vi "Lidar Finder_OLD.vi"(3 "Stop":bool, 5 "VISA resource name":refnum<visa-resource-name>="Hukuyo") -> (0 "Objects":cluster{i32, i32}[](array[cluster]), 1 "Widest Object":cluster{i32, i32}, 2 "Where to Point":i32)   [LabVIEW 2014]
uses:
  <instrlib>/Hokuyo URG Series/Public/Initialize-Standard.vi
  <instrlib>/Hokuyo URG Series/Hokuyo URG Series.lvlib
panel:
  in  "Tab Control":enum32{"Raw Data", "Clean Data"}(tab)
  out "Data Aquired":picture
  out "Object Graph":i32[](graph)
  out "Edges":i32[](graph)
  out "Blinky LIDAR  Running":bool
  in  "polar attributes (hidden)":T1={"maximum"=30000.0, "minimum"=0.0, "clip to min"=FALSE, "log?(F)"=TRUE, "grid color"=6710886, "plot color"=65280, "fmt and prec"={"format"=enum."Decimal", "precision"=0}, "visible section"=8} {"minimum" format="%0.2f"; "maximum" format="%0.2f"}
  in  "Grid Color":u32(colorbox)=11776947
  in  "Plot Color":u32(colorbox)=14422272
  in  "Max (m)":dbl=1.0
  in  "End Point":dbl=40.0
  in  "Start Point":dbl=-50.0
  in  "Cluster Count":dbl=1.0
  in  "Encoding Width":u16(ring)=3 items=["2 Byte"=2, "3 Byte"=3]
  # "click here to run"
  # "Hokuyo LIDAR Example"
  # "Plot in mm"
  # "start at-50"
  # "start at 40"
  # "Start with 1.0 m"
  # "Hokuyo plugged in?"
  # "Location"
  # "Width"
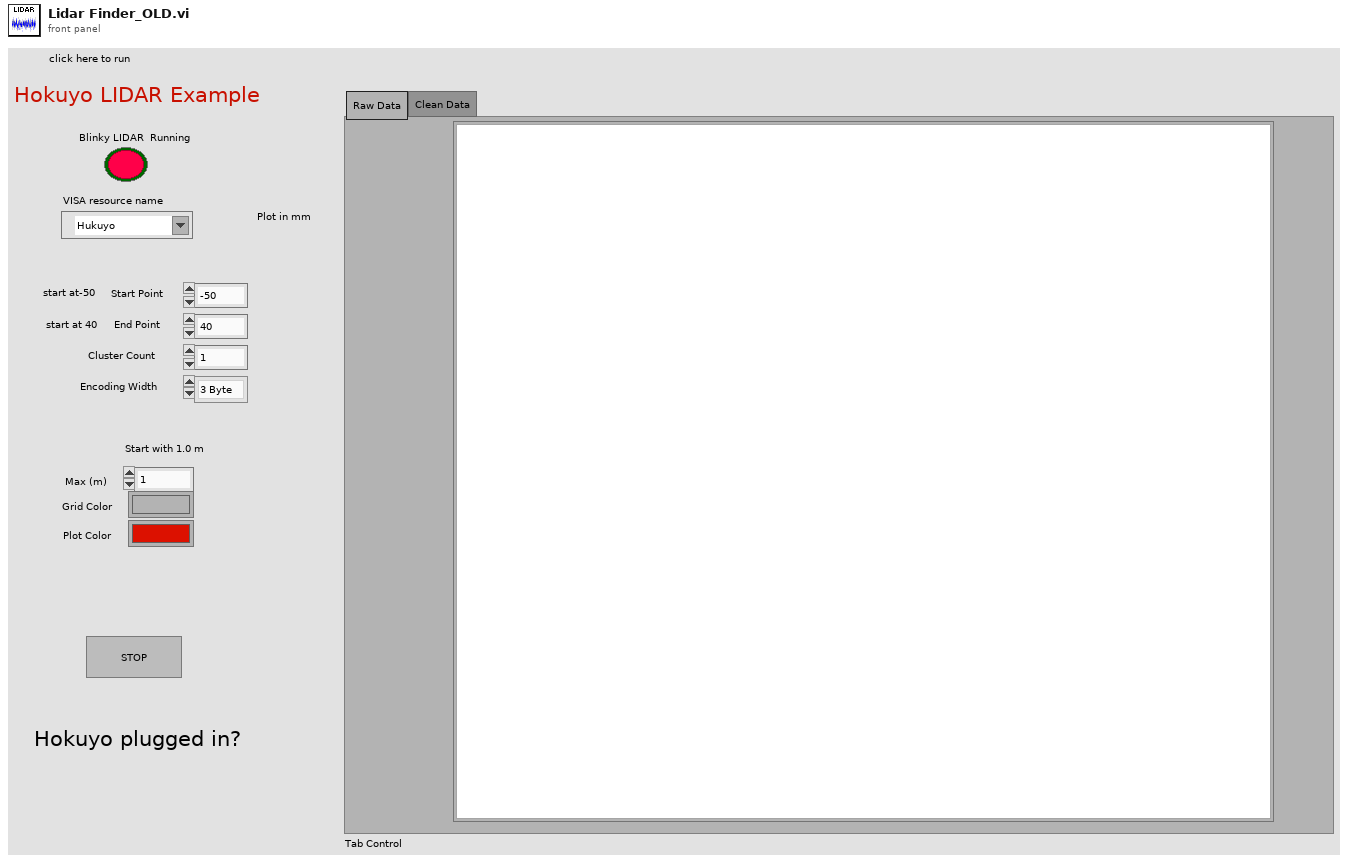
[diagram p1: front panel]
types:
  T1 = cluster{"maximum":dbl, "minimum":dbl, "clip to min":bool, "log?(F)":bool, "grid color":u32, "plot color":u32, "fmt and prec":cluster{"format":enum8{"Decimal", "Scientific", "Engineering", "Binary", "Octal", "Hex"}, "precision":u8}, "visible section":u16}
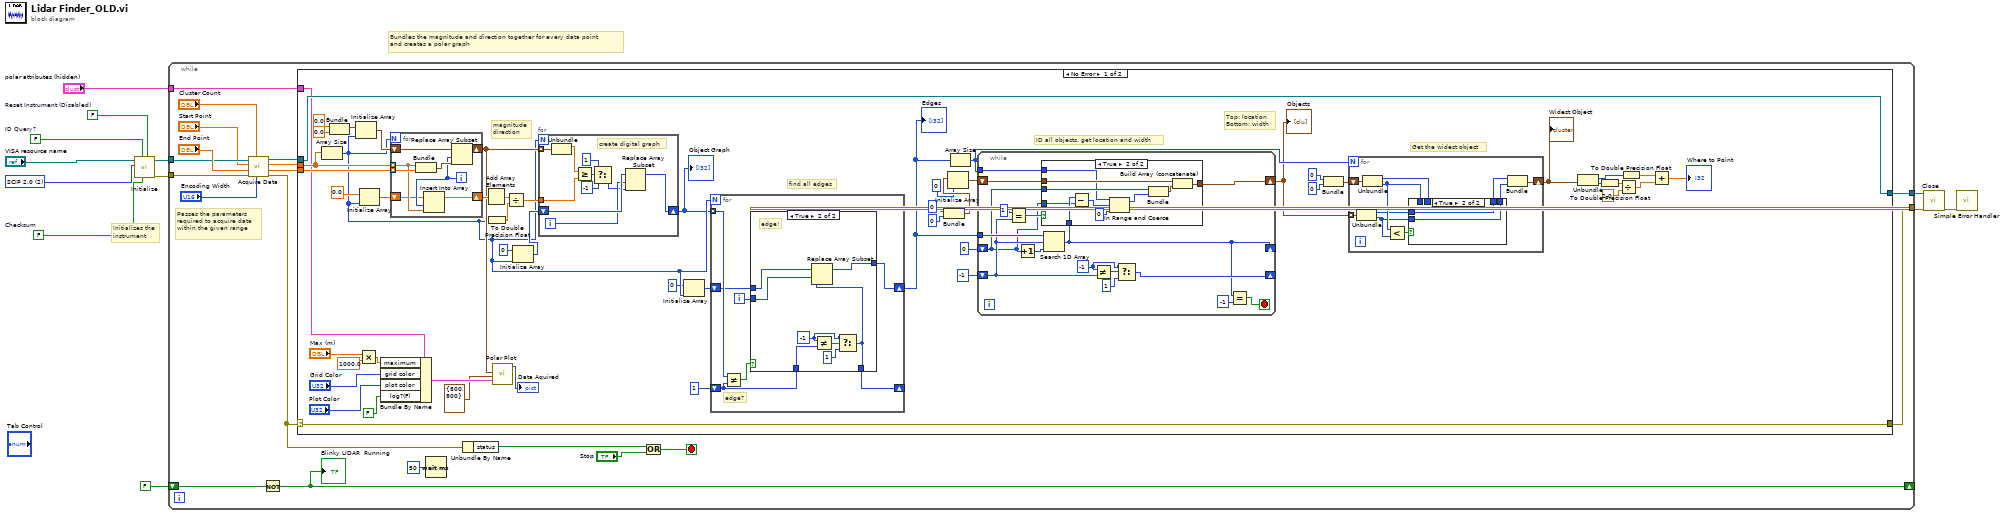
[diagram p0: block diagram]
diagram:
  w10 = FALSE  # Checksum
  w8 = FALSE  # ID Query?
  w6 = u32 2 items=["Convert to Latest", "SCIP 1.1", "SCIP 2.0"] ("Protocol")
  w7 = FALSE  # Reset Instrument (Disabled)
  # "Bundles the magnitude and direction together for every data point\nand creates a polar graph"
  # "Initializes the instrument"
  n1 = call-poly <instrlib>:"Initialize.vi"("Reset? (F: No)"=w7, "Checksum (Disabled)"=w10, "ID Query? (Enabled)"=w8, "Protocol (2: SCIP 2.0)"=w6, "VISA resource name"="VISA resource name") -> ("error out"=w3:errorcluster, "VISA resource name out"=w4:refnum<visa-resource-name>)  [unwired: 5 in]
  n2 = while {
    tunnel: w4 -> [w20]
    tunnel: [w31] -> w12
    tunnel: [w30] -> w5
    tunnel: w3 -> [w19]
    tunnel: "polar attributes (hidden)" -> [w18]
    shift-right: [w14] -> _
    shift-left: FALSE -> [w15]
    stop <- w27 stop-if-true
    # "Passes the parameters\nrequired to acquire data\nwithin the given range"
    n3 = call <instrlib>:"Acquire Data.vi"("Data Encoding Width (3 Byte)"="Encoding Width", "Cluster Count (1)"="Cluster Count", "error in (no error)"=w19, "End Point (120°)"="End Point", "Start Point (-120°)"="Start Point", "VISA resource name"=w20) -> ("error out"=w23:errorcluster, "Direction"=w24:dbl[], "Magnitude"=w25:dbl[], "VISA resource name out"=w26:refnum<visa-resource-name>)  [unwired: 2 in]
    n4 = Not(x=w15) -> (.not. x?=w14:bool)
    "Blinky LIDAR  Running" <- w14
    n5 = case shown="No Error" w23 {
      selector: w23 -> [w82 w162]
      tunnel: [w82 w162] -> w31
      tunnel: w26 -> [w83 w161]
      tunnel: [w83 w161] -> w30
      tunnel: w25 -> [w77 _]
      tunnel: w24 -> [w76 _]
      tunnel: w18 -> [w74 _]
      frame No Error {
        # "Get the widest object"
        # "Top: location\nBottom: width"
        # "find all edges"
        # "ID all objects, get location and width"
        # "magnitude\ndirection"
        n6 = Array Size(array=w77) -> (size(s)=w56:i32)
        n7 = Bundle(0.0, 0.0) -> (w79:cluster{dbl, dbl})  [unwired: 1 in]
        n8 = Initialize Array(w79, w56) -> (w78:cluster{dbl, dbl}[])
        n9 = Multiply(x="Max (m)", y=1000.0) -> (x*y=w70:dbl)
        n10 = Initialize Array(0.0, w56) -> (w65:dbl[])
        n11 = Bundle By Name(cluster=w74, "maximum"=w70, "grid color"="Grid Color", "plot color"="Plot Color", "log?(F)"=FALSE) -> (w75:T1)
        n12 = for {
          N: w56 -> [_]
          shift-right: [w158] -> w61
          shift-left: w78 -> [w159]
          tunnel: w77 -> [w155] mode=indexing
          tunnel: w76 -> [w160] mode=indexing
          shift-right: [w153] -> w64
          shift-left: w65 -> [w154]
          i -> [w156]
          n13 = Bundle(w155, w160) -> (w157:cluster{dbl, dbl})  [unwired: 1 in]
          n14 = Insert Into Array(array=w154, index=w156, new element=w155) -> (w153:dbl[])
          n15 = Replace Array Subset(array=w159, new element=w157, index=w156) -> (w158:cluster{dbl, dbl}[])
        }
        n16 = Add Array Elements(numeric array=w64) -> (sum=w63:dbl)
        n17 = To Double Precision Float(number=w56) -> (double precision float=w62:dbl)
        n18 = call <vilib>:"Polar Plot.vi"("polar attributes"=w75, "dimensions (w,h)"=cluster{"width":i16, "height":i16} {"width"=800, "height"=800}, "data array [mag, phase (deg)]"=w61) -> ("new picture"=→"Data Aquired":picture)  [unwired: 8 in]
        n19 = Divide(x=w63, y=w62) -> (x/y=w60:dbl)
        n20 = Initialize Array(0, w56) -> (w59:i32[])
        n21 = for {
          N: w56 -> [_]
          tunnel: w61 -> [w152] mode=indexing
          tunnel: w60 -> [w150]
          shift-right: [w147] -> w53
          shift-left: w59 -> [w149]
          i -> [w148]
          # "create digital graph"
          n22 = Unbundle(w152) -> (w151:dbl)  [unwired: 1 out]
          n23 = Greater Or Equal?(x=w151, y=w150) -> (x >= y?=w145:bool)
          n24 = Select(t=1, s=w145, f=-1) -> (s? t:f=w146:i32)
          n25 = Replace Array Subset(array=w149, new element=w146, index=w148) -> (w147:i32[])
        }
        "Object Graph" <- w53
        n26 = Initialize Array(0, w56) -> (w54:i32[])
        n27 = for {
          N: w56 -> [_]
          shift-right: [w130] -> _
          shift-left: 1 -> [w129]
          tunnel: w53 -> [w131] mode=indexing
          shift-right: [w126] -> w45
          shift-left: w54 -> [w128]
          i -> [w127]
          # "edge?"
          n28 = Not Equal?(x=w131, y=w129) -> (x != y?=w132:bool)
          n29 = case shown="True" w132 {
            tunnel: [w134 w136] -> w130
            tunnel: w129 -> [w134 w142]
            tunnel: w128 -> [w133 w138]
            tunnel: w127 -> [_ w137]
            tunnel: [w133 w135] -> w126
            frame False {
              # "no edge"
            }
            frame True {
              w140 = -1
              # "edge!"
              n30 = Not Equal?(x=w140, y=w142) -> (x != y?=w141:bool)
              n31 = Select(t=w140, s=w141, f=1) -> (s? t:f=w136:i32)
              n32 = Replace Array Subset(array=w138, new element=w136, index=w137) -> (w135:i32[])
            }
          }
        }
        "Edges" <- w45
        n33 = Bundle(0, 0) -> (w49:cluster{i32, i32})  [unwired: 1 in]
        n34 = Initialize Array(w49, 0) -> (w50:cluster{i32, i32}[])
        n35 = Array Size(array=w45) -> (size(s)=w44:i32)
        n36 = while {
          tunnel: w45 -> [w112]
          shift-right: [w108] -> _
          shift-left: -1 -> [w103]
          shift-right: [w105] -> _
          shift-left: 0 -> [w100]
          shift-right: [w107] -> w40
          shift-left: w50 -> [w106]
          tunnel: w44 -> [w99]
          stop <- w114 stop-if-true
          w110 = -1
          n37 = Equal?(x=1, y=w103) -> (x = y?=w102:bool)
          n38 = Increment(x=w100) -> (x+1=w101:i32)
          n39 = Search 1D Array(1D array=w112, element=w103, start index (0)=w101) -> (index of element=w105:i32)
          n40 = case shown="True" w102 {
            tunnel: [w115 w125] -> w107
            tunnel: w106 -> [w115 w124]
            tunnel: w105 -> [_ w122]
            tunnel: w100 -> [_ w121]
            tunnel: w100 -> [_ w120]
            tunnel: w99 -> [_ w119]
            frame False {
            }
            frame True {
              n41 = Subtract(x=w122, y=w121) -> (x-y=w118:i32)
              n42 = In Range and Coerce(upper limit=w119, x=w118, lower limit=0) -> (coerced(x)=w117:i32)  [unwired: 1 out]
              n43 = Bundle(w120, w117) -> (w123:cluster{i32, i32})  [unwired: 1 in]
              n44 = Build Array (concatenate)(w124, w123) -> (w125:cluster{i32, i32}[])
            }
          }
          n45 = Not Equal?(x=w110, y=w103) -> (x != y?=w109:bool)
          n46 = Select(t=w110, s=w109, f=1) -> (s? t:f=w108:i32)
          n47 = Equal?(x=w105, y=-1) -> (x = y?=w114:bool)
        }
        "Objects" <- w40
        n48 = Bundle(0, 0) -> (w41:cluster{i32, i32})  [unwired: 1 in]
        n49 = for {
          N: w44 -> [_]
          shift-right: [w93] -> w39
          shift-left: w41 -> [w94]
          tunnel: w40 -> [w89] mode=indexing
          n50 = Unbundle(w89) -> (w86:i32, w85:i32)
          n51 = Unbundle(w94) -> (w91:i32, w87:i32)
          n52 = Less?(x=w87, y=w85) -> (x < y?=w88:bool)
          n53 = case shown="True" w88 {
            tunnel: [w96 w98] -> w92
            tunnel: w91 -> [w96 _]
            tunnel: [w95 w97] -> w90
            tunnel: w87 -> [w95 _]
            tunnel: w86 -> [_ w98]
            tunnel: w85 -> [_ w97]
            frame False {
            }
            frame True {
            }
          }
          n54 = Bundle(w92, w90) -> (w93:cluster{i32, i32})  [unwired: 1 in]
        }
        "Widest Object" <- w39
        n55 = Unbundle(w39) -> (w33:i32, w37:i32)
        n56 = To Double Precision Float(number=w37) -> (double precision float=w36:dbl)
        n57 = Divide(x=w36, y=2.0) -> (x/y=w34:dbl)
        n58 = To Double Precision Float(number=w33) -> (double precision float=w32:dbl)
        n59 = Add(x=w32, y=w34) -> (x+y=→"Where to Point":dbl)
      }
      frame Error {
      }
    }
    n60 = Wait (ms)(milliseconds to wait=u32 50) -> ()  [unwired: 1 out]
    n61 = Unbundle By Name(w23) -> ("status"=w29:bool)
    n62 = Or(x=w29, y="Stop") -> (x .or. y?=w27:bool)
  }
  n63 = call <instrlib>:"Close.vi"("error in (no error)"=w12, "VISA resource name"=w5) -> ("error out"=w9:errorcluster)  [unwired: 9 in]
  n64 = call <vilib>:"Simple Error Handler.vi"("error in (no error)"=w9) -> ()  [unwired: 4 in, 5 out]
